vi "_wmg_ImpSpecDivided@.vi"(1 "Input":string="1@110@2@105@3@103;1@90@2@95@3@97") -> (0 "Output":string[][](array[string]))   [LabVIEW 2011]
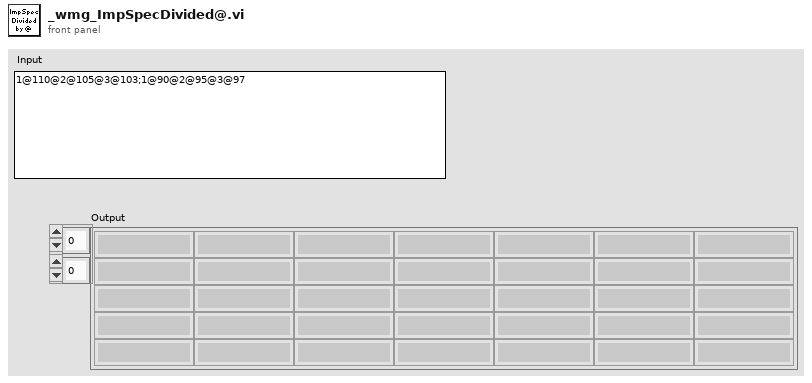
[diagram p1: front panel]
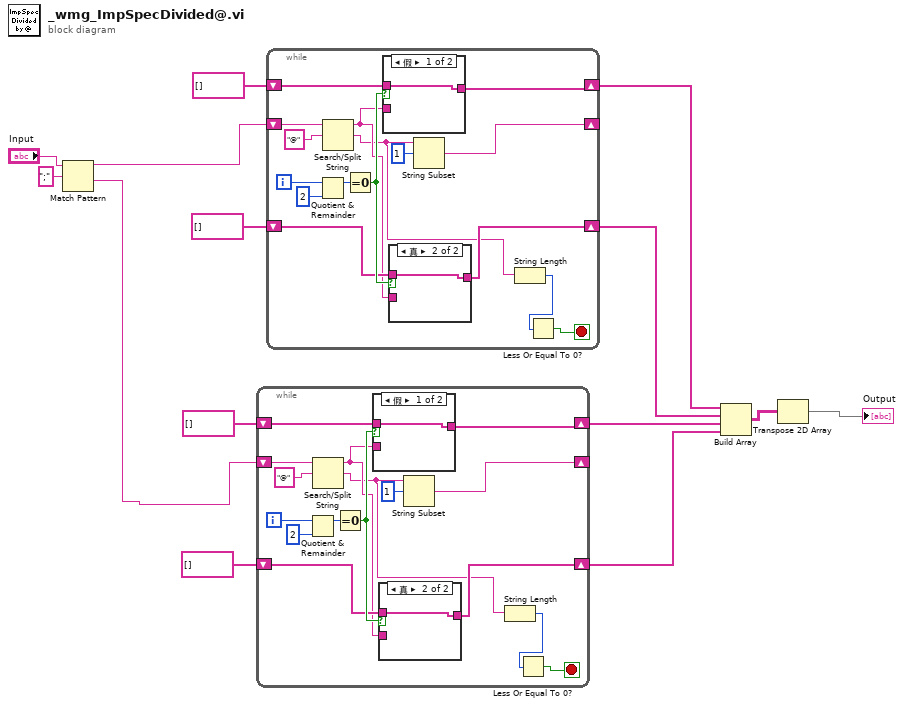
[diagram p0: block diagram]
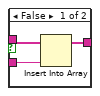
[diagram p2: hidden frame]
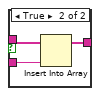
[diagram p3: hidden frame]
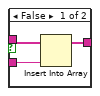
[diagram p4: hidden frame]
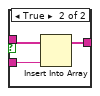
[diagram p5: hidden frame]
diagram:
  n1 = Match Pattern(string="Input", regular expression=";" ("正则表达式")) -> (before substring=w12:string, after substring=w7:string)  [unwired: 1 in, 2 out]
  n2 = while {
    shift-right: [w18] -> _
    shift-left: w7 -> [w30]
    shift-right: [w25] -> w4
    shift-left: string[] [] -> [w26]
    shift-right: [w20] -> w3
    shift-left: string[] [] -> [w22]
    i -> [w28]
    stop <- w16 stop-if-true
    n3 = Quotient & Remainder(x=w28, y=2) -> (x-y*floor(x/y)=w24:i32)  [unwired: 1 out]
    n4 = Search/Split String(string=w30, search string/char (-)="@" ("搜索字符串/字符(-)")) -> (substring before match=w21:string, match + rest of string=w17:string)  [unwired: 1 in, 1 out]
    n5 = Equal To 0?(x=w24) -> (x = 0?=w23:bool)
    n6 = case shown="假" w23 {
      tunnel: w26 -> [w35 w38]
      tunnel: [w35 w37] -> w25
      tunnel: w21 -> [_ w36]
      frame False {
      }
      frame True {
        n7 = Insert Into Array(array=w38, new element=w36) -> (w37:string[])  [unwired: 1 in]
      }
    }
    n8 = case shown="真" w23 {
      tunnel: w22 -> [w33 w34]
      tunnel: [w32 w34] -> w20
      tunnel: w21 -> [w31 _]
      frame False {
        n9 = Insert Into Array(array=w33, new element=w31) -> (w32:string[])  [unwired: 1 in]
      }
      frame True {
      }
    }
    n10 = String Subset(string=w17, offset (0)=1 ("偏移量(0)")) -> (substring=w18:string)  [unwired: 1 in]
    n11 = String Length(string=w17) -> (length=w15:i32)
    n12 = Less Or Equal To 0?(x=w15) -> (x <= 0?=w16:bool)
  }
  n13 = while {
    shift-right: [w42] -> _
    shift-left: w12 -> [w54]
    shift-right: [w49] -> w6
    shift-left: string[] [] -> [w50]
    shift-right: [w44] -> w5
    shift-left: string[] [] -> [w46]
    i -> [w52]
    stop <- w40 stop-if-true
    n14 = Quotient & Remainder(x=w52, y=2) -> (x-y*floor(x/y)=w48:i32)  [unwired: 1 out]
    n15 = Search/Split String(string=w54, search string/char (-)="@" ("搜索字符串/字符(-)")) -> (substring before match=w45:string, match + rest of string=w41:string)  [unwired: 1 in, 1 out]
    n16 = Equal To 0?(x=w48) -> (x = 0?=w47:bool)
    n17 = case shown="假" w47 {
      tunnel: w50 -> [w59 w62]
      tunnel: [w59 w61] -> w49
      tunnel: w45 -> [_ w60]
      frame False {
      }
      frame True {
        n18 = Insert Into Array(array=w62, new element=w60) -> (w61:string[])  [unwired: 1 in]
      }
    }
    n19 = case shown="真" w47 {
      tunnel: w46 -> [w57 w58]
      tunnel: [w56 w58] -> w44
      tunnel: w45 -> [w55 _]
      frame False {
        n20 = Insert Into Array(array=w57, new element=w55) -> (w56:string[])  [unwired: 1 in]
      }
      frame True {
      }
    }
    n21 = String Subset(string=w41, offset (0)=1 ("偏移量(0)")) -> (substring=w42:string)  [unwired: 1 in]
    n22 = String Length(string=w41) -> (length=w39:i32)
    n23 = Less Or Equal To 0?(x=w39) -> (x <= 0?=w40:bool)
  }
  n24 = Build Array(w6, w5, w4, w3) -> (w2:string[][])
  n25 = Transpose 2D Array(2D array=w2) -> (transposed array=→"Output":string[][])
